vi "Initialize.vi"(6 "optional":variant, 8 "error in":errorcluster, 11 "DMA_Read in":refnum<class "DMA_Read.lvclass">) -> (0 "error out":errorcluster, 3 "Node*":refnum<data-value>)   [LabVIEW 2013, in "DMA_Read.lvclass"]
doc: "Initializes a node. Makes a data value reference of the node, sets the selfNode, and output the data value reference."
uses:
  DMA_Read.lvclass
  xCE/xceNode/xceNode.lvclass
  xCE/xceDataNode/xceDataNode.lvclass
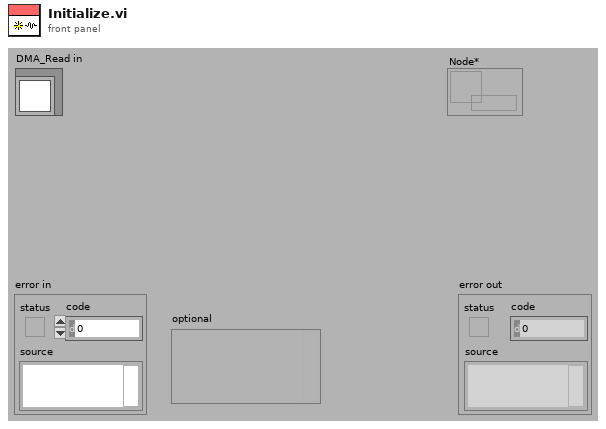
[diagram p1: front panel]
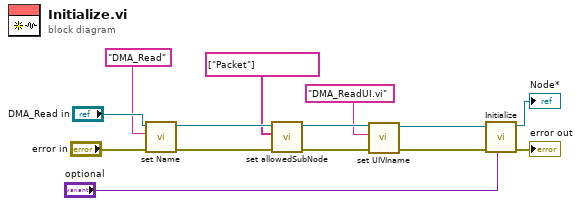
[diagram p0: block diagram]
diagram:
  n1 = call "set Name.vi"("error in (no error)"="error in", "Name"="DMA_Read", "xceDataNode in"="DMA_Read in") -> ("error out"=w6:errorcluster, "xceDataNode out"=w8:refnum<class "DMA_Read.lvclass">)  [unwired: 7 in]
  n2 = call "set allowedSubNode.vi"("error in (no error)"=w6, "Allowed subNode[]"=string[] ["Packet"], "xceDataNode in"=w8) -> ("error out"=w4:errorcluster, "xceDataNode out"=w5:refnum<class "DMA_Read.lvclass">)  [unwired: 7 in]
  n3 = call "set UIVIname.vi"("error in (no error)"=w4, "UI VI name"="DMA_ReadUI.vi", "xceDataNode in"=w5) -> ("error out"=w1:errorcluster, "xceDataNode out"=w2:refnum<class "DMA_Read.lvclass">)  [unwired: 7 in]
  n4 = call-parent "Initialize.vi"("optional"="optional", "error in"=w1, "xceDataNode in"=w2) -> ("error out"=→"error out":errorcluster, "Node*"=→"Node*":refnum<data-value>)  [unwired: 7 in]
